vi "MKS_PDR2000_open.vi"(8 "error in (no error)":errorcluster, 11 "PDR2000 COM port":refnum<visa-resource-name>) -> (0 "error out":errorcluster, 3 "PDR2000 COM port out":refnum<visa-resource-name>)   [LabVIEW 2019]
uses:
  <vilib>/Instr/_visa.llb/VISA Open Access Mode.ctl
  <vilib>/Instr/_visa.llb/VISA Configure Serial Port (Instr).vi
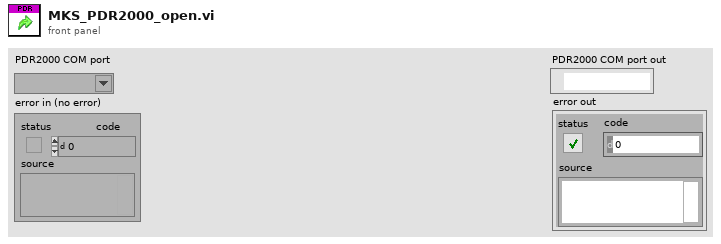
[diagram p1: front panel]
types:
  T1 = typedef "VISA Open Access Mode.ctl" = u32
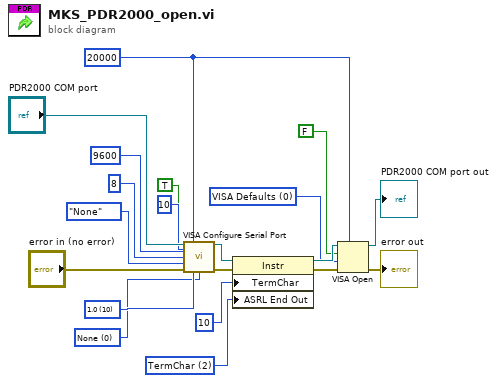
[diagram p0: block diagram]
diagram:
  w5 = T1 0 items=["VISA Defaults"=0, "Exclusive Lock"=1, "Load Configured Settings"=4] ("Access Mode")
  w8 = u16 2 items=["None", "Last Bit", "TermChar", "Break"] ("Serial Settings:End Mode for Writes")
  w3 = u32 20000 ("timeout (10sec)")
  w14 = u16 0 items=["None", "XON/XOFF", "RTS/CTS", "XON/XOFF & RTS/CTS", "DTR/DSR", "XON/XOFF & DTR/DSR"] ("flow control (0:none)")
  w15 = u16 10 items=["1.0"=10, "1.5"=15, "2.0"=20] ("stop bits (10: 1 bit)")
  n1 = call-poly "VISA Configure Serial Port"("VISA resource name"="PDR2000 COM port", "timeout (10sec)"=w3, "termination char\n(0xA = '\\n' = LF)"=u8 10 ("termination char\n(0xA = '\\n' = LF)"), "Enable Termination\nChar (T)"=TRUE ("Enable Termination\nChar (T)"), "baud rate (9600)"=u32 9600, "data bits (8)"=u16 8, "parity (0:none)"=enum16{"None", "Odd", "Even", "Mark", "Space"}."None", "error in (no error)"="error in (no error)", "stop bits (10: 1 bit)"=w15, "flow control (0:none)"=w14) -> ("VISA resource name out"=w11:refnum<visa-resource-name>, "error out"=w10:errorcluster)  [unwired: 4 in]
  n2 = property class="Instr"(reference=w11, error in=w10, "TermChar"=u8 10 ("Message Based Settings:Termination Character"), "ASRL End Out"=w8) -> (reference out=w7:refnum<visa-resource-name>, error out=w6:errorcluster)
  n3 = VISA Open(timeout (0)=w3, duplicate session (F)=FALSE, access mode=w5, error in (no error)=w6, VISA resource name=w7) -> (VISA resource name=→"PDR2000 COM port out":refnum<visa-resource-name>, error out=→"error out":errorcluster)
